vi "test read timing source.vi"() -> (0 "no error":errorcluster)   [LabVIEW 2013, in "TBM Tests.lvlib"]
uses:
  TBM Tests.lvlib
  runtime/TBM module execution interface.lvclass
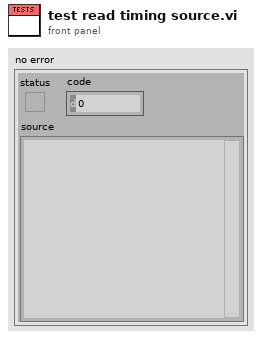
[diagram p1: front panel]
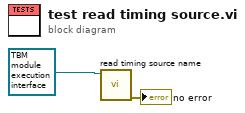
[diagram p0: block diagram]
diagram:
  n1 = call-dynamic "read timing source name.vi"("module in"=refnum<class "TBM module execution interface.lvclass"> refnum ("module")) -> ("error out"=→"no error":errorcluster)  [unwired: 8 in, 2 out]
